vi "Client Complete Streaming Call.vi"(8 "error in":errorcluster, 10 "Cancel All Reads (F)":bool, 11 "Call ID in":T2) -> (0 "error out":errorcluster, 1 "errorDetails":T1)   [LabVIEW 2019, in "grpc-lvsupport.lvlib"]
doc: "Set \"Cancel All Reads\" to true to end all pending reads and ignore any outstanding data from server that hasn't been read yet. If this setting is false, all server data must be read before the client can close the stream."
uses:
  grpc-lvsupport.lvlib
  Shared/Any.ctl
  Shared/grpcId.ctl
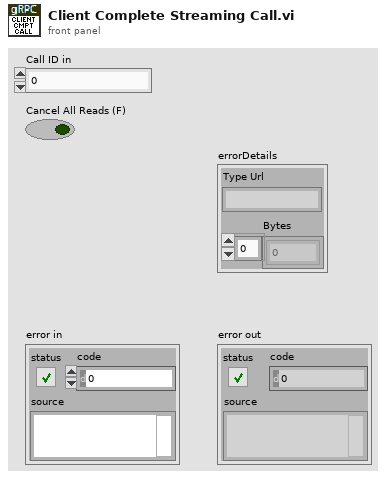
[diagram p1: front panel]
types:
  T1 = typedef "grpc-lvsupport.lvlib/Any.ctl" = cluster{"Type Url":string, "Bytes":u8[]}
  T2 = typedef "grpc-lvsupport.lvlib/grpcId.ctl" = u64
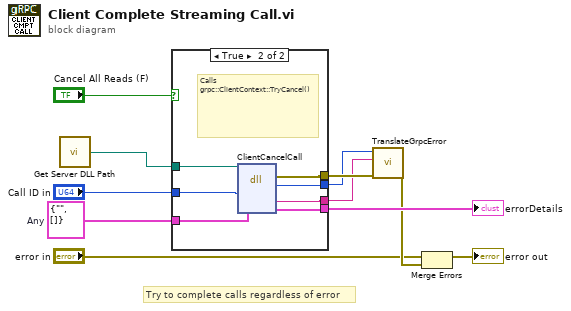
[diagram p0: block diagram]
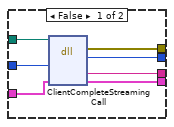
[diagram p2: hidden frame]
diagram:
  w8 = T1 {"Type Url"="", "Bytes"=[]}  # Any
  # "Try to complete calls regardless of error"
  n1 = call "Get Server DLL Path.vi"() -> ("server dll path"=w9:path)
  n2 = case shown="True" "Cancel All Reads (F)" {
    tunnel: [w18 w22] -> w11
    tunnel: "Call ID in" -> [w17 w24]
    tunnel: w9 -> [w16 w25]
    tunnel: w8 -> [w15 w23]
    tunnel: [w14 w19] -> w7
    tunnel: [w13 w20] -> w6
    tunnel: [w12 w21] -> w5
    frame False {
      n3 = dll-call lib="?" fn="ClientCompleteStreamingCall"(path in=w16, "ClientId"=w17, "errorDetails"=w15) -> (error out=w18:errorcluster, "return type"=w12:i32, "errorMessage"=w13:string, "errorDetails"=w14:T1)  [unwired: 4 in, 1 out]
    }
    frame True {
      # "Calls \ngrpc::ClientContext::TryCancel()"
      n4 = dll-call lib="?" fn="ClientCancelCall"(path in=w25, "ClientId"=w24, "errorDetails"=w23) -> (error out=w22:errorcluster, "return type"=w21:i32, "errorMessage"=w20:string, "errorDetails"=w19:T1)  [unwired: 4 in, 1 out]
    }
  }
  "errorDetails" <- w7
  n5 = call "TranslateGrpcError.vi"("error in"=w11, "Error Message"=w6, "Error Code"=w5) -> ("error out"=w4:errorcluster)  [unwired: 8 in]
  n6 = Merge Errors("error in", w4) -> (→"error out":errorcluster)
